vi "getPixelMapping.vi"(11 "Key String IN":string) -> (1 "Rectangle":T1, 2 "Y_Pixel Map":i32[](array[numeric]), 3 "X_Pixel Map":i32[](array[numeric]), 4 "y.pixels":i32, 5 "Calibration Available?":bool, 6 "x.pixels":i32)   [LabVIEW 2012]
uses:
  GFG/GFGstringGet.vi
  GFG/GFGbooleanGet.vi
  <vilib>/Utility/config.llb/Read Key (String).vi
  <vilib>/Utility/config.llb/NI_LVConfig.lvlib
  GFG/GFG library.lvlib
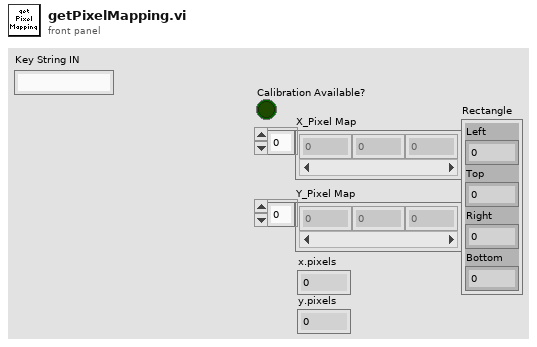
[diagram p1: front panel]
types:
  T1 = cluster{"Left":i32, "Top":i32, "Right":i32, "Bottom":i32}
  T2 = typedef "NI_LVConfig.lvlib/Config Data RefNum.ctl" = refnum<k1>
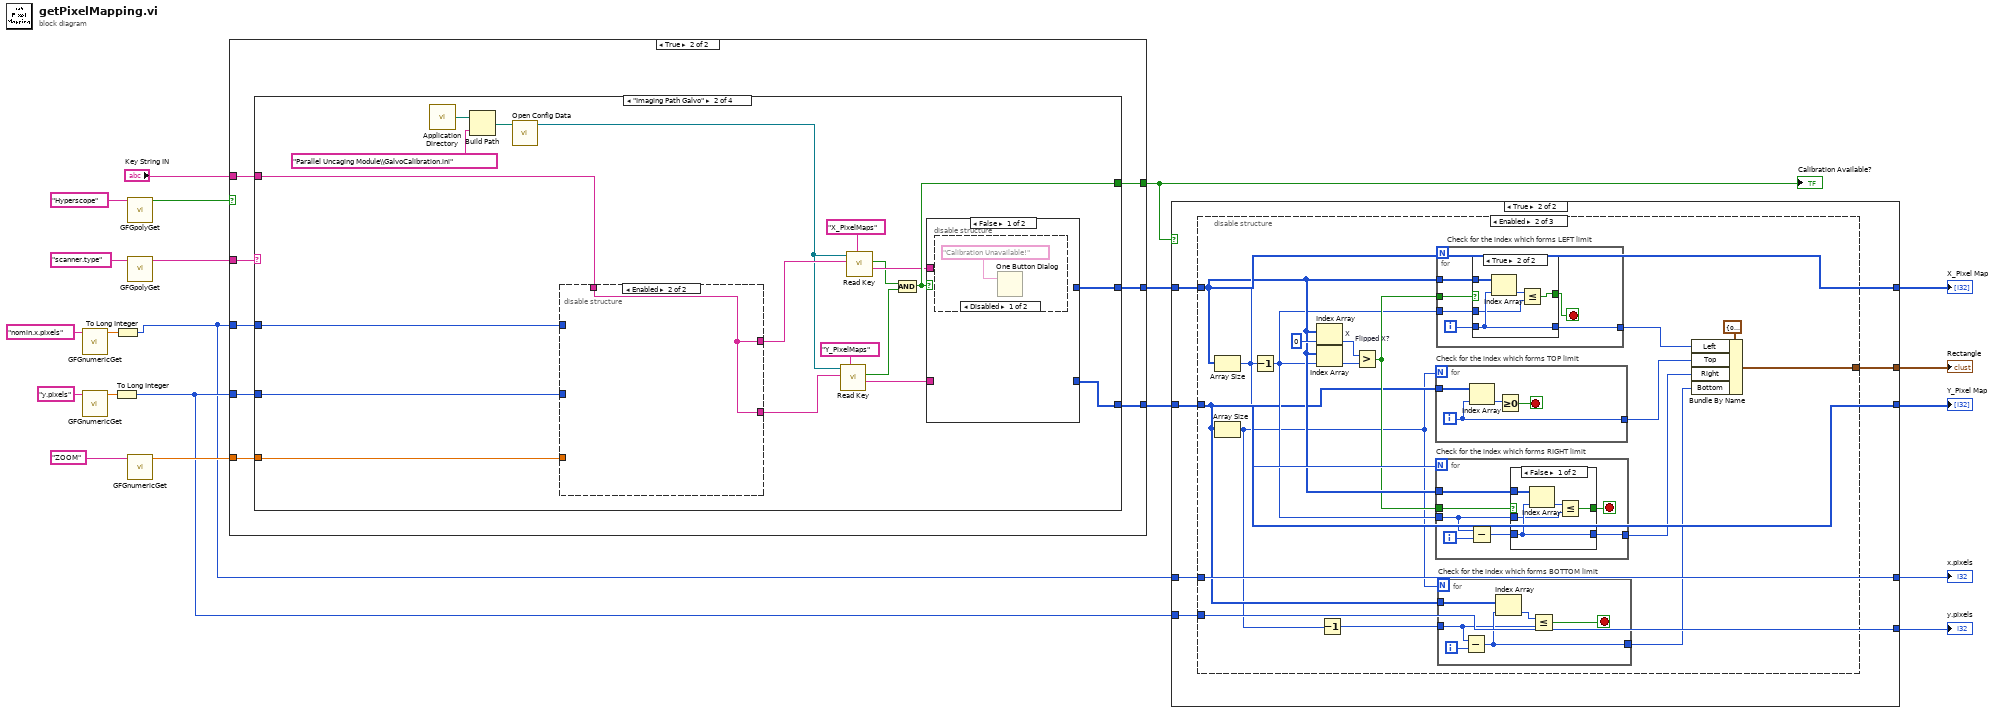
[diagram p0: block diagram]
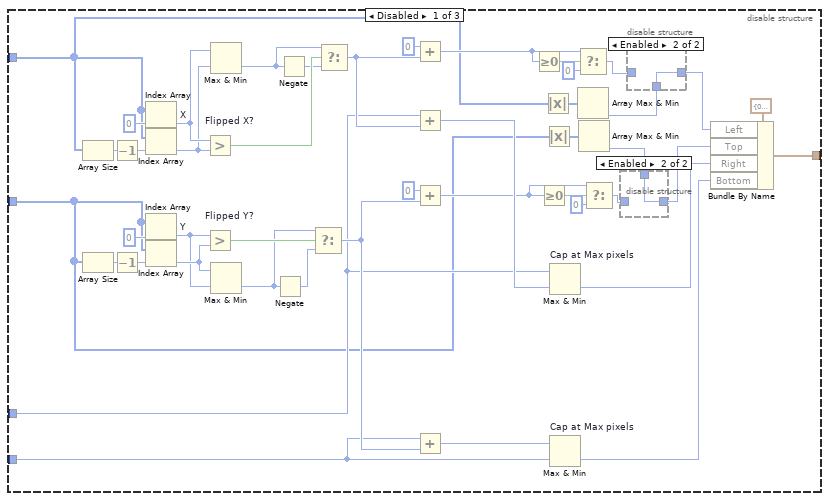
[diagram p3: hidden frame]
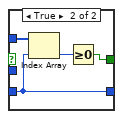
[diagram p6: hidden frame]
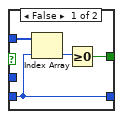
[diagram p7: hidden frame]
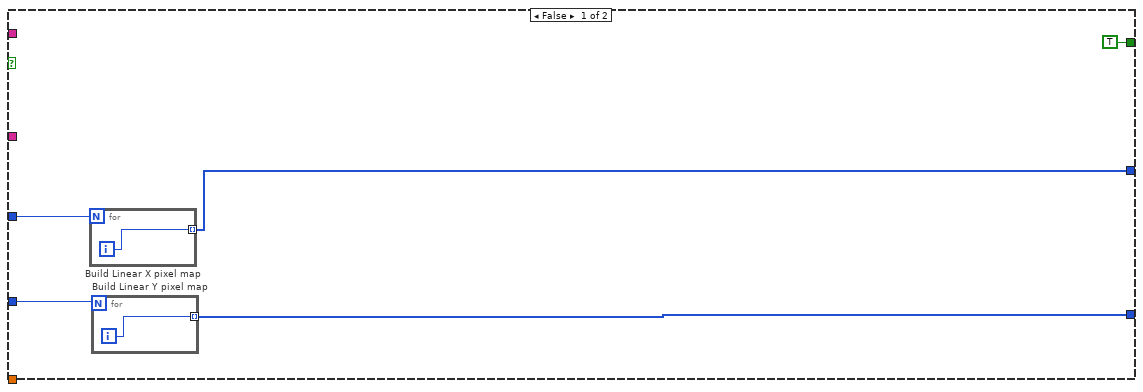
[diagram p9: hidden frame]
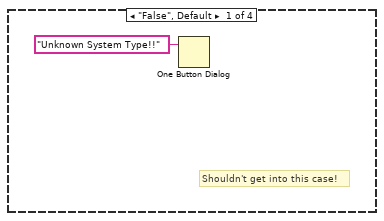
[diagram p10: hidden frame]
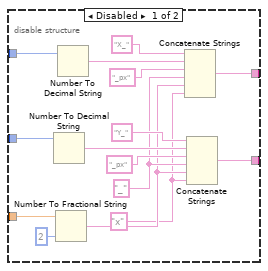
[diagram p11: hidden frame]
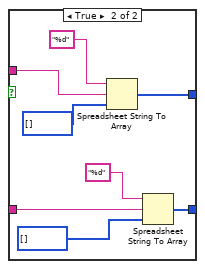
[diagram p13: hidden frame]
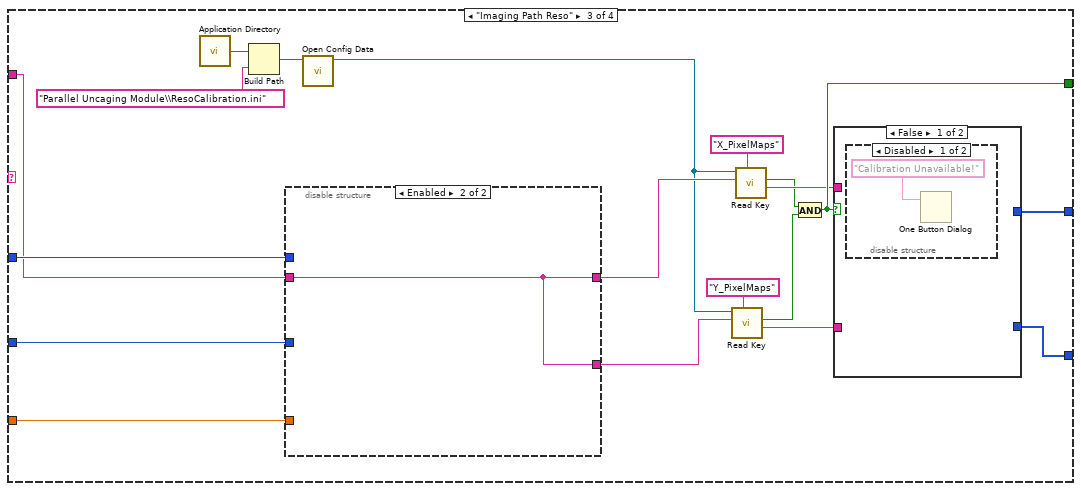
[diagram p14: hidden frame]
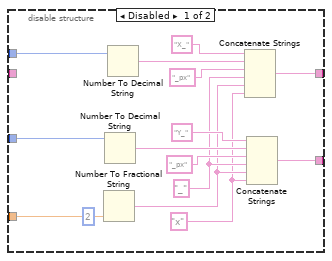
[diagram p15: hidden frame]
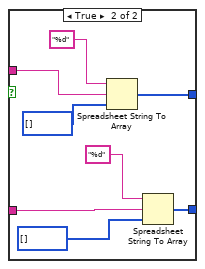
[diagram p17: hidden frame]
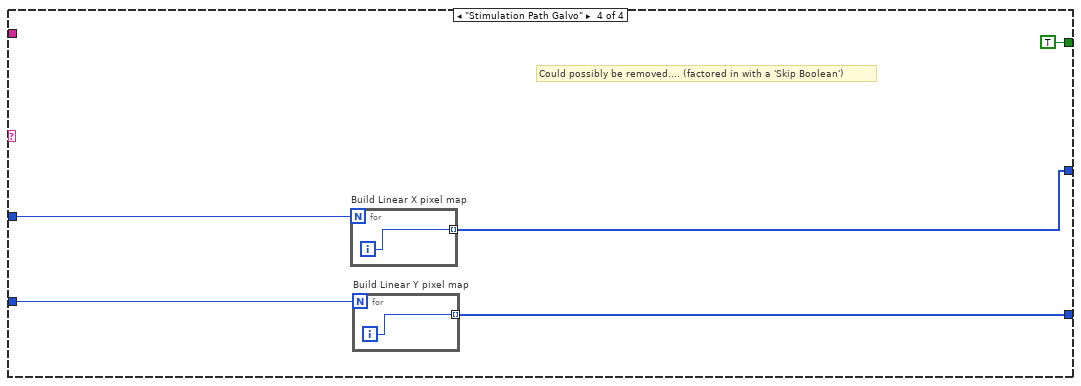
[diagram p18: hidden frame]
diagram:
  n1 = call "GFGnumericGet.vi"("Variable Name in"="nomin.x.pixels") -> ("Numeric"=w2:dbl)  [unwired: 8 in, 2 out]
  n2 = call "GFGnumericGet.vi"("Variable Name in"="y.pixels") -> ("Numeric"=w1:dbl)  [unwired: 8 in, 2 out]
  n3 = To Long Integer(number=w1) -> (32bit integer=w6:i32)
  n4 = To Long Integer(number=w2) -> (32bit integer=w5:i32)
  n5 = call-poly "GFGpolyGet.vi"("Variable Name in"="Hyperscope") -> ("Boolean Value OUT"=w19:bool)  [unwired: 9 in, 1 out]
  n6 = call-poly "GFGpolyGet.vi"("Variable Name in"="scanner.type") -> ("String"=w18:string)  [unwired: 9 in, 1 out]
  n7 = call "GFGnumericGet.vi"("Variable Name in"="ZOOM") -> ("Numeric"=w12:dbl)  [unwired: 8 in, 2 out]
  n8 = case shown="True" w19 {
    tunnel: w5 -> [w26 w36]
    tunnel: [w24 w35] -> w14
    tunnel: w6 -> [w25 w34]
    tunnel: [w23 w33] -> w15
    tunnel: w12 -> [_ w32]
    tunnel: [TRUE w31] -> w17
    tunnel: w18 -> [_ w30]
    tunnel: "Key String IN" -> [_ w29]
    frame False {
      n9 = for "Build Linear X pixel map" {
        N: w26 -> [_]
        tunnel: [w28] -> w24 mode=indexing
        i -> [w28]
      }
      n10 = for "Build Linear Y pixel map" {
        N: w25 -> [_]
        tunnel: [w27] -> w23 mode=indexing
        i -> [w27]
      }
    }
    frame True {
      n11 = case shown="\"Imaging Path Galvo\"" w30 {
        tunnel: w36 -> [_ w40 w100 w130]
        tunnel: [_ w56 w99 w127] -> w35
        tunnel: w34 -> [_ w39 w98 w129]
        tunnel: [_ w55 w97 w128] -> w33
        tunnel: w32 -> [_ w54 w96 _]
        tunnel: [_ w53 w95 TRUE] -> w31
        tunnel: w29 -> [_ w38 w82 _]
        frame "False", Default {
          # "Shouldn't get into this case!"
          n12 = One Button Dialog(message="Unknown System Type!!") -> ()  [unwired: 1 in, 1 out]
        }
        frame "Imaging Path Galvo" {
          n13 = call <vilib>:"Application Directory.vi"() -> ("Application Directory"=w52:path)
          n14 = Build Path(base path=w52, name or relative path="Parallel Uncaging Module\\GalvoCalibration.ini") -> (appended path=w51:path)
          n15 = call <vilib>:"Open Config Data.vi"("configuration file path"=w51) -> ("refnum"=w45:T2)  [unwired: 8 in, 2 out]
          n16 = disable-structure shown="Enabled" {
            disable-tunnel: w54 -> [w71 _]
            disable-tunnel: [w67 w72] -> w49
            disable-tunnel: [w63 w72] -> w46
            disable-tunnel: w40 -> [w58 _]
            disable-tunnel: w39 -> [w57 _]
            disable-tunnel: w38 -> [_ w72]
            frame Disabled {
              w59 = "x" ("string")
              w61 = "_" ("string")
              n17 = Number To Decimal String(number=w57) -> (decimal integer string=w65:string)  [unwired: 1 in]
              n18 = Number To Fractional String(number=w71, precision (6)=i16 2) -> (F-format string=w60:string)  [unwired: 2 in]
              n19 = Number To Decimal String(number=w58) -> (decimal integer string=w69:string)  [unwired: 1 in]
              n20 = Concatenate Strings("X_" ("string"), w69, "_px" ("string"), w61, w60, w59) -> (w67:string)
              n21 = Concatenate Strings("Y_" ("string"), w65, "_px" ("string"), w61, w60, w59) -> (w63:string)
            }
            frame Enabled {
            }
          }
          n22 = call-poly <vilib>:"Read Key.vi"("section"="Y_PixelMaps", "key"=w46, "refnum"=w45) -> ("value"=w42:string, "found?"=w43:bool)  [unwired: 5 in, 2 out]
          n23 = call-poly <vilib>:"Read Key.vi"("section"="X_PixelMaps", "key"=w49, "refnum"=w45) -> ("value"=w48:string, "found?"=w44:bool)  [unwired: 5 in, 2 out]
          n24 = And(x=w44, y=w43) -> (x .and. y?=w53:bool)
          n25 = case shown="False" w53 {
            tunnel: w48 -> [_ w79]
            tunnel: [_ w78] -> w56
            tunnel: w42 -> [_ w75]
            tunnel: [_ w74] -> w55
            frame False {
              n26 = disable-structure shown="Disabled" {
                frame Disabled {
                  n27 = One Button Dialog(message="Calibration Unavailable!") -> ()  [unwired: 1 in, 1 out]
                }
                frame Enabled {
                }
              }
            }
            frame True {
              n28 = Spreadsheet String To Array(format string="%d", spreadsheet string=w79, array type (2D Dbl)=i32[] []) -> (array=w78:i32[])  [unwired: 1 in]
              n29 = Spreadsheet String To Array(format string="%d", spreadsheet string=w75, array type (2D Dbl)=i32[] []) -> (array=w74:i32[])  [unwired: 1 in]
            }
          }
        }
        frame "Imaging Path Reso" {
          n30 = call <vilib>:"Application Directory.vi"() -> ("Application Directory"=w94:path)
          n31 = Build Path(base path=w94, name or relative path="Parallel Uncaging Module\\ResoCalibration.ini") -> (appended path=w93:path)
          n32 = disable-structure shown="Enabled" {
            disable-tunnel: w100 -> [w115 _]
            disable-tunnel: w98 -> [w114 _]
            disable-tunnel: w96 -> [w113 _]
            disable-tunnel: [w109 w116] -> w91
            disable-tunnel: [w105 w116] -> w88
            disable-tunnel: w82 -> [_ w116]
            frame Disabled {
              w101 = "x" ("string")
              w103 = "_" ("string")
              n33 = Number To Fractional String(number=w113, precision (6)=i16 2) -> (F-format string=w102:string)  [unwired: 2 in]
              n34 = Number To Decimal String(number=w114) -> (decimal integer string=w107:string)  [unwired: 1 in]
              n35 = Number To Decimal String(number=w115) -> (decimal integer string=w111:string)  [unwired: 1 in]
              n36 = Concatenate Strings("X_" ("string"), w111, "_px" ("string"), w103, w102, w101) -> (w109:string)
              n37 = Concatenate Strings("Y_" ("string"), w107, "_px" ("string"), w103, w102, w101) -> (w105:string)
            }
            frame Enabled {
            }
          }
          n38 = call <vilib>:"Open Config Data.vi"("configuration file path"=w93) -> ("refnum"=w87:T2)  [unwired: 8 in, 2 out]
          n39 = call-poly <vilib>:"Read Key.vi"("section"="Y_PixelMaps", "key"=w88, "refnum"=w87) -> ("value"=w84:string, "found?"=w85:bool)  [unwired: 5 in, 2 out]
          n40 = call-poly <vilib>:"Read Key.vi"("section"="X_PixelMaps", "key"=w91, "refnum"=w87) -> ("value"=w90:string, "found?"=w86:bool)  [unwired: 5 in, 2 out]
          n41 = And(x=w86, y=w85) -> (x .and. y?=w95:bool)
          n42 = case shown="False" w95 {
            tunnel: w90 -> [_ w123]
            tunnel: [_ w122] -> w99
            tunnel: w84 -> [_ w119]
            tunnel: [_ w118] -> w97
            frame False {
              n43 = disable-structure shown="Disabled" {
                frame Disabled {
                  n44 = One Button Dialog(message="Calibration Unavailable!") -> ()  [unwired: 1 in, 1 out]
                }
                frame Enabled {
                }
              }
            }
            frame True {
              n45 = Spreadsheet String To Array(format string="%d", spreadsheet string=w123, array type (2D Dbl)=i32[] []) -> (array=w122:i32[])  [unwired: 1 in]
              n46 = Spreadsheet String To Array(format string="%d", spreadsheet string=w119, array type (2D Dbl)=i32[] []) -> (array=w118:i32[])  [unwired: 1 in]
            }
          }
        }
        frame "Stimulation Path Galvo" {
          # "Could possibly be removed.... (factored in with a 'Skip Boolean')"
          n47 = for "Build Linear X pixel map" {
            N: w130 -> [_]
            tunnel: [w132] -> w127 mode=indexing
            i -> [w132]
          }
          n48 = for "Build Linear Y pixel map" {
            N: w129 -> [_]
            tunnel: [w131] -> w128 mode=indexing
            i -> [w131]
          }
        }
      }
    }
  }
  "Calibration Available?" <- w17
  n49 = case shown="True" w17 {
    tunnel: w14 -> [w134 w138]
    tunnel: w15 -> [w133 w137]
    tunnel: [_ w141] -> w16
    tunnel: w6 -> [w135 w139]
    tunnel: w5 -> [w136 w140]
    tunnel: [w136 w140] -> w11
    tunnel: [w135 w139] -> w10
    tunnel: [w134 w138] -> w8
    tunnel: [w133 w137] -> w9
    frame False {
    }
    frame True {
      n50 = disable-structure shown="Enabled" {
        disable-tunnel: [w182 w203 _] -> w141
        disable-tunnel: w140 -> [w153 _ _]
        disable-tunnel: w139 -> [w152 _ _]
        disable-tunnel: w138 -> [w151 w197 _]
        disable-tunnel: w137 -> [w148 w193 _]
        frame Disabled {
          n51 = Array Size(array=w151) -> (size(s)=w175:i32)
          n52 = Array Size(array=w148) -> (size(s)=w173:i32)
          n53 = Decrement(x=w175) -> (x-1=w174:i32)
          n54 = Decrement(x=w173) -> (x-1=w172:i32)
          n55 = Index Array "X"(array=w151, index=0) -> (element=w159:i32)
          n56 = Index Array(array=w151, index=w174) -> (element=w158:i32)
          n57 = Index Array "Y"(array=w148, index=0) -> (element=w155:i32)
          n58 = Index Array(array=w148, index=w172) -> (element=w156:i32)
          n59 = Greater? "Flipped X?"(x=w159, y=w158) -> (0:w170:bool)
          n60 = Greater? "Flipped Y?"(x=w155, y=w156) -> (0:w167:bool)
          n61 = Max & Min(x=w159, y=w158) -> (min(x,y)=w157:i32)  [unwired: 1 out]
          n62 = Max & Min(x=w156, y=w155) -> (min(x,y)=w154:i32)  [unwired: 1 out]
          n63 = Negate(x=w154) -> (-x=w166:i32)
          n64 = Negate(x=w157) -> (-x=w169:i32)
          n65 = Select(t=w154, s=w167, f=w166) -> (s? t:f=w165:i32)
          n66 = Select(t=w157, s=w170, f=w169) -> (s? t:f=w168:i32)
          n67 = Add(x=0 ("f"), y=w168) -> (x+y=w163:i32)
          n68 = Add(x=w153, y=w168) -> (x+y=w164:i32)
          n69 = Add(x=0 ("f"), y=w165) -> (x+y=w161:i32)
          n70 = Add(x=w152, y=w165) -> (x+y=w162:i32)
          n71 = Greater Or Equal To 0?(x=w163) -> (x >= 0?=w180:bool)
          n72 = Greater Or Equal To 0?(x=w161) -> (x >= 0?=w176:bool)
          n73 = Absolute Value(x=w151) -> (abs(x)=w150:i32[])
          n74 = Absolute Value(x=w148) -> (abs(x)=w149:i32[])
          n75 = Max & Min "Cap at Max pixels"(x=w153, y=w164) -> (min(x,y)=w181:i32)  [unwired: 1 out]
          n76 = Max & Min "Cap at Max pixels"(x=w162, y=w152) -> (min(x,y)=w178:i32)  [unwired: 1 out]
          n77 = Select(t=w163, s=w180, f=0) -> (s? t:f=w147:i32)
          n78 = Array Max & Min(array=w150) -> (min index (indices)=w145:i32)  [unwired: 3 out]
          n79 = Array Max & Min(array=w149) -> (min index (indices)=w142:i32)  [unwired: 3 out]
          n80 = Select(t=w161, s=w176, f=0) -> (s? t:f=w144:i32)
          n81 = disable-structure shown="Enabled" {
            disable-tunnel: w144 -> [w186 _]
            disable-tunnel: [w186 w187] -> w143
            disable-tunnel: w142 -> [_ w187]
            frame Disabled {
            }
            frame Enabled {
            }
          }
          n82 = disable-structure shown="Enabled" {
            disable-tunnel: w147 -> [w188 _]
            disable-tunnel: [w188 w189] -> w146
            disable-tunnel: w145 -> [_ w189]
            frame Disabled {
            }
            frame Enabled {
            }
          }
          n83 = Bundle By Name(cluster=T1 {"Left"=0, "Top"=0, "Right"=0, "Bottom"=0} ("Rectangle"), "Left"=w146, "Top"=w143, "Right"=w181, "Bottom"=w178) -> (w182:T1)
        }
        frame Enabled {
          n84 = Array Size(array=w197) -> (size(s)=w198:i32)
          n85 = Array Size(array=w193) -> (size(s)=w192:i32)
          n86 = Decrement(x=w198) -> (x-1=w195:i32)
          n87 = Index Array "X"(array=w197, index=0) -> (element=w202:i32)
          n88 = Index Array(array=w197, index=w195) -> (element=w201:i32)
          n89 = Decrement(x=w192) -> (x-1=w191:i32)
          n90 = Greater? "Flipped X?"(x=w202, y=w201) -> (0:w196:bool)
          n91 = for "Check for the index which forms TOP limit" {
            N: w192 -> [_]
            tunnel: w193 -> [w231]
            tunnel: [w229] -> w199
            i -> [w229]
            stop <- w230 stop-if-true
            n92 = Index Array(array=w231, index=w229) -> (element=w228:i32)
            n93 = Greater Or Equal To 0?(x=w228) -> (x >= 0?=w230:bool)
          }
          n94 = for "Check for the index which forms RIGHT limit" {
            N: w198 -> [_]
            tunnel: w197 -> [w217]
            tunnel: w196 -> [w218]
            tunnel: w195 -> [w212]
            tunnel: [w215] -> w194
            i -> [w214]
            stop <- w216 stop-if-true
            n95 = Subtract(x=w212, y=w214) -> (x-y=w213:i32)
            n96 = case shown="False" w218 {
              tunnel: w217 -> [w223 w225]
              tunnel: [w222 w226] -> w216
              tunnel: [w220 w224] -> w215
              tunnel: w213 -> [w220 w224]
              tunnel: w212 -> [w219 _]
              frame False {
                n97 = Index Array(array=w223, index=w220) -> (element=w221:i32)
                n98 = Less Or Equal?(x=w221, y=w219) -> (x <= y?=w222:bool)
              }
              frame True {
                n99 = Index Array(array=w225, index=w224) -> (element=w227:i32)
                n100 = Greater Or Equal To 0?(x=w227) -> (x >= 0?=w226:bool)
              }
            }
          }
          n101 = for "Check for the index which forms LEFT limit" {
            N: w198 -> [_]
            tunnel: w197 -> [w236]
            tunnel: w196 -> [w237]
            tunnel: w195 -> [w232]
            tunnel: [w233] -> w200
            i -> [w235]
            stop <- w234 stop-if-true
            n102 = case shown="True" w237 {
              tunnel: w236 -> [w238 w245]
              tunnel: w235 -> [w239 w246]
              tunnel: [w240 w244] -> w234
              tunnel: [w239 w246] -> w233
              tunnel: w232 -> [_ w242]
              frame False {
                n103 = Index Array(array=w238, index=w239) -> (element=w241:i32)
                n104 = Greater Or Equal To 0?(x=w241) -> (x >= 0?=w240:bool)
              }
              frame True {
                n105 = Index Array(array=w245, index=w246) -> (element=w243:i32)
                n106 = Less Or Equal?(x=w243, y=w242) -> (x <= y?=w244:bool)
              }
            }
          }
          n107 = for "Check for the index which forms BOTTOM limit" {
            N: w192 -> [_]
            tunnel: w193 -> [w211]
            tunnel: [w208] -> w190
            tunnel: w191 -> [w207]
            i -> [w209]
            stop <- w206 stop-if-true
            n108 = Subtract(x=w207, y=w209) -> (x-y=w208:i32)
            n109 = Index Array(array=w211, index=w208) -> (element=w210:i32)
            n110 = Less Or Equal?(x=w210, y=w207) -> (x <= y?=w206:bool)
          }
          n111 = Bundle By Name(cluster=T1 {"Left"=0, "Top"=0, "Right"=0, "Bottom"=0} ("Rectangle"), "Left"=w200, "Top"=w199, "Right"=w194, "Bottom"=w190) -> (w203:T1)
        }
        frame Disabled {
        }
      }
    }
  }
  "X_Pixel Map" <- w8
  "Y_Pixel Map" <- w9
  "Rectangle" <- w16
  "y.pixels" <- w10
  "x.pixels" <- w11
